vi "Write Shutoff Valve State.vi"(8 "error in":errorcluster, 9 "Obersve or Ignore Safe State":u16(ring) items=["Observe"=0, "Ignore"=256], 10 "Valve State":T1, 11 "MB_TCP session in":refnum<class "MB_Master_TCP.lvclass">) -> (0 "error out":errorcluster, 2 "(hi.lo)":u32, 3 "MB session out":refnum<class "MB_Master_TCP.lvclass">)   [LabVIEW 2024, in "Bronkhorst Flexi-Flow ModbusTCP API.lvlib"]
uses:
  Bronkhorst Flexi-Flow ModbusTCP API.lvlib
  <vilib>/Plasmionique/MB Master/MB_Master_TCP/MB_Master_TCP.lvclass
  C:/Program Files/National Instruments/LabVIEW 2025/vi.lib/Plasmionique/MB Master/MB_Master/MB_Master.lvclass
  Valve State--enum.ctl
  <vilib>/Plasmionique/MB Master/MB Master.lvlib
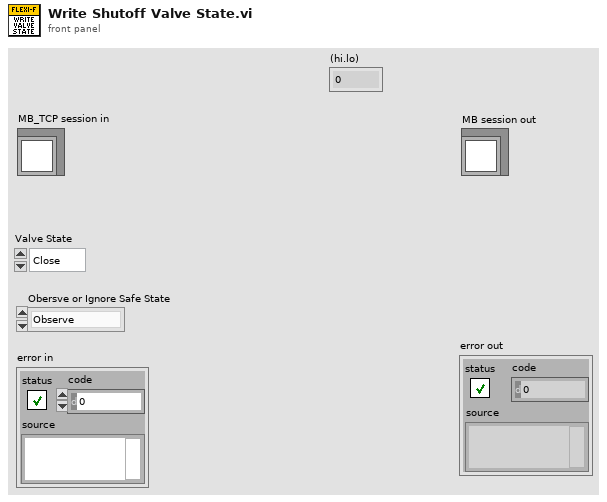
[diagram p1: front panel]
types:
  T1 = typedef "Bronkhorst Flexi-Flow ModbusTCP API.lvlib/Valve State--enum.ctl" = enum16{"Close", "Open"}
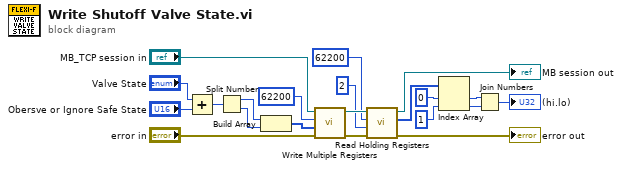
[diagram p0: block diagram]
diagram:
  n1 = Add(x="Valve State", y="Obersve or Ignore Safe State") -> (x+y=w18:u16)
  n2 = Split Number(x=w18) -> (hi(x)=w17:u8, lo(x)=w16:u8)
  n3 = Build Array(w17, w16) -> (w15:u8[])
  n4 = call <vilib>:"Write Multiple Registers.vi"("error in (no error)"="error in", "values"=w15, "starting address"=u16 62200, "MB session in"="MB_TCP session in") -> ("error out"=w12:errorcluster, "MB session out"=w13:refnum<class "MB_Master_TCP.lvclass">)  [unwired: 6 in]
  n5 = call <vilib>:"Read Holding Registers.vi"("error in (no error)"=w12, "quantity"=u16 2, "starting address"=u16 62200, "MB session in"=w13) -> ("error out"=→"error out":errorcluster, "Registers"=w9:u16[], "MB session out"=→"MB session out":refnum<class "MB_Master_TCP.lvclass">)  [unwired: 5 in]
  n6 = Index Array(array=w9, index #1=0 ("index"), index #2=1 ("index")) -> (element #1=w6:u16, element #2=w5:u16)
  n7 = Join Numbers(hi=w6, lo=w5) -> ((hi.lo)=→"(hi.lo)":u32)
